vi "Drive Motor TXRX.vi"(6 "Configuration":T3={"Accelerometer Bias"={"X (m/s)"=0.0, "Y (m/s)"=0.0, "Z (m/s)"=0.0}, "Gyroscope Bias"={"X (m/s)"=0.0, "Y (m/s)"=0.0, "Z (m/s)"=0.0}, "Steering Motor Gear Ratio"=611.0, "Steering Pully Gear Ratio"=1.0, "Steering Encoder CPR"=500.0, "Steering Motor Max RPM"=4000.0, "Wheelbase (m)"=1.12, "Fork Angle (rad)"=1.3, "Balancing Controller"={"Kp (/s)"=0.0, "Kd (1)"=0.0}, "Max Allowed Steering Angle (rad)"=0.7, "Task Periods"={"Emergency Stop (us)"=0, "IMU (us)"=0, "Steering Motor Encoder (us)"=0, "State Estimator (us)"=0, "Balancing Controller (us)"=0, "GNSS (us)"=0, "Logging (us)"=0, "Drive Motor (us)"=0}, "Drive Motor Gear Ratio"=0.7}, 8 "Controller Data In":refnum<data-value>, 9 "Angular Speed (rad/s)":dbl, 10 "Drive Motor Handle In":T2, 11 "Error In":errorcluster) -> (0 "Controller Data Out":refnum<data-value>, 1 "Drive Motor Data":T1, 2 "Drive Motor Handle Out":T2, 3 "Error Out":errorcluster)   [LabVIEW 2021]
uses:
  Drive Motor Handle.ctl
  Configuration/Configuration.ctl
  Drive Motor Data.ctl
  Logging/Controller Data.ctl
  Steering Motor/Steering Motor Data.ctl
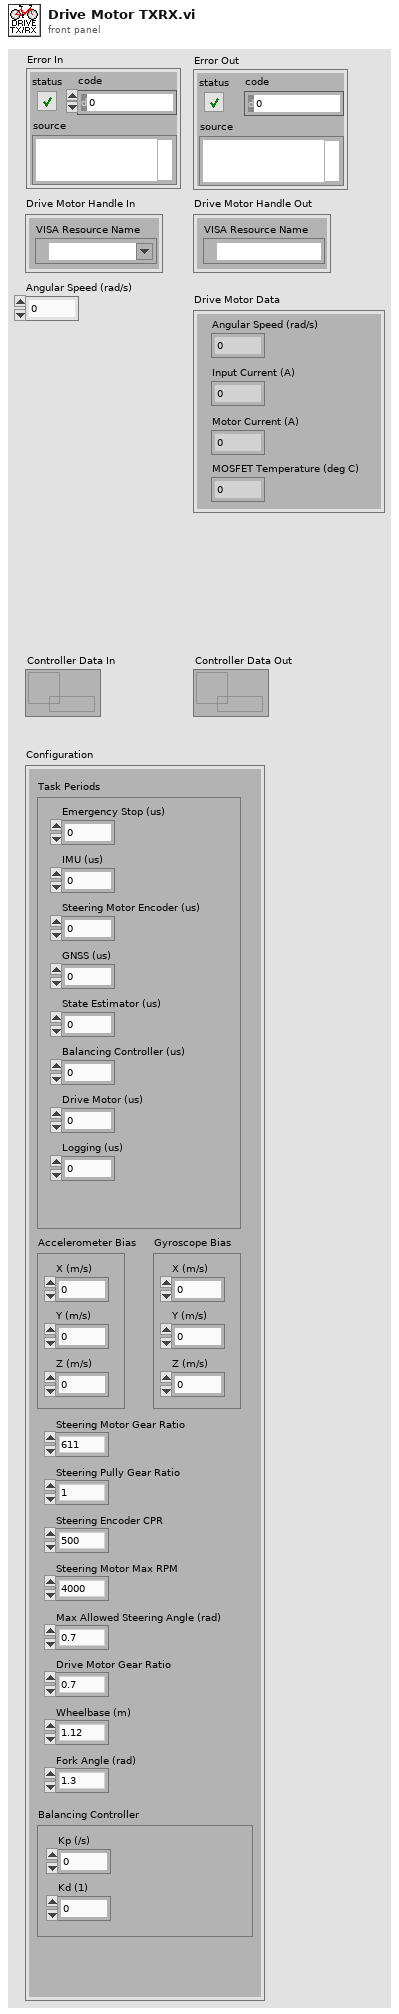
[diagram p1: front panel]
types:
  T1 = typedef "Drive Motor Data.ctl" = cluster{"Angular Speed (rad/s)":dbl, "Input Current (A)":dbl, "Motor Current (A)":dbl, "MOSFET Temperature (deg C)":dbl}
  T2 = typedef "Drive Motor Handle.ctl" = cluster{"VISA Resource Name":refnum<visa-resource-name>}
  T3 = typedef "Configuration.ctl" = cluster{"Accelerometer Bias":cluster{"X (m/s)":dbl, "Y (m/s)":dbl, "Z (m/s)":dbl}, "Gyroscope Bias":cluster{"X (m/s)":dbl, "Y (m/s)":dbl, "Z (m/s)":dbl}, "Steering Motor Gear Ratio":dbl, "Steering Pully Gear Ratio":dbl, "Steering Encoder CPR":dbl, "Steering Motor Max RPM":dbl, "Wheelbase (m)":dbl, "Fork Angle (rad)":dbl, "Balancing Controller":cluster{"Kp (/s)":dbl, "Kd (1)":dbl}, "Max Allowed Steering Angle (rad)":dbl, "Task Periods":cluster{"Emergency Stop (us)":i64, "IMU (us)":i64, "Steering Motor Encoder (us)":i64, "State Estimator (us)":i64, "Balancing Controller (us)":i64, "GNSS (us)":i64, "Logging (us)":i64, "Drive Motor (us)":i64}, "Drive Motor Gear Ratio":dbl}
  T4 = typedef "Controller Data.ctl" = cluster{"Drive Motor Data":T1, "Steering Motor Data":T5}
  T5 = typedef "Steering Motor Data.ctl" = cluster{"PWM":dbl, "Steering Angle Rate (rad/s)":dbl}
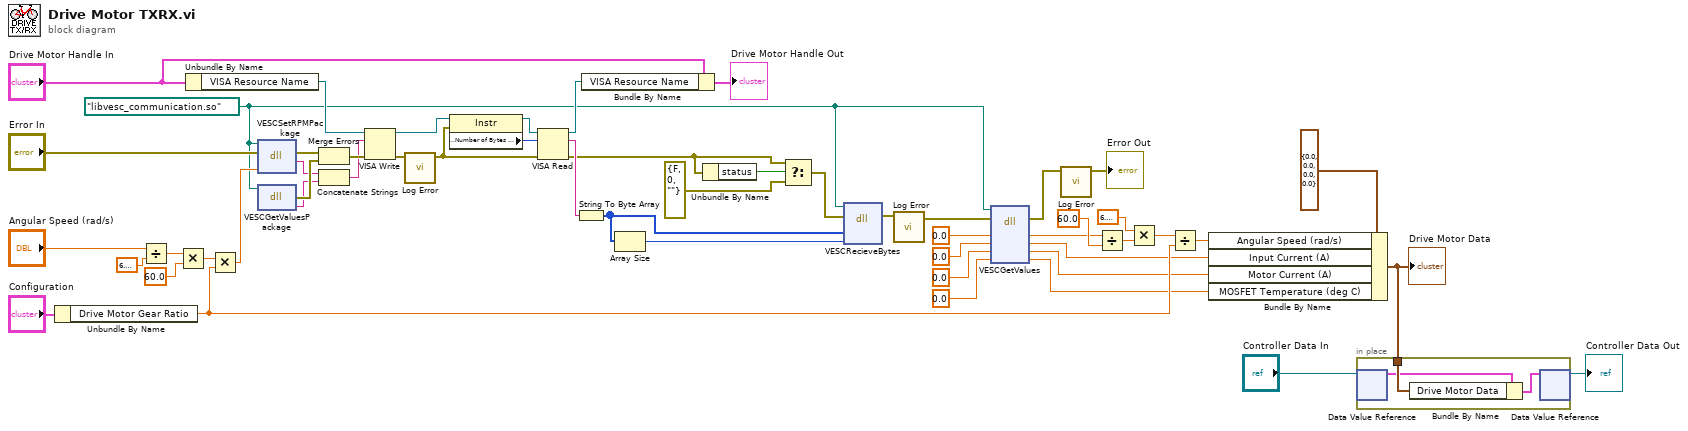
[diagram p0: block diagram]
diagram:
  w36 = path "libvesc_communication.so" ("path in")
  n1 = Unbundle By Name("Configuration") -> ("Drive Motor Gear Ratio"=w35:dbl)
  n2 = Divide(x="Angular Speed (rad/s)", y=6.283185307179586) -> (x/y=w50:dbl)
  n3 = Multiply(x=w50, y=60.0) -> (x*y=w48:dbl)
  n4 = Unbundle By Name("Drive Motor Handle In") -> ("VISA Resource Name"=w42:refnum<visa-resource-name>)
  n5 = Multiply(x=w48, y=w35) -> (x*y=w47:dbl)
  n6 = dll-call lib="?" fn="VESCSetRPMPackage"(path in=w36, error in="Error In", "RPM"=w47) -> (error out=w41:errorcluster, "Package"=w3:string)  [unwired: 2 in, 1 out]
  n7 = dll-call lib="?" fn="VESCGetValuesPackage"(path in=w36) -> (error out=w40:errorcluster, "Package"=w2:string)  [unwired: 2 in, 1 out]
  n8 = Merge Errors(w41, w40) -> (w39:errorcluster)
  n9 = Concatenate Strings(w3, w2) -> (w1:string)
  n10 = VISA Write(VISA resource name=w42, write buffer=w1, error in (no error)=w39) -> (VISA resource name out=w38:refnum<visa-resource-name>, error out=w45:errorcluster)  [unwired: 1 out]
  n11 = call "Log Error.vi"("Error In"=w45) -> ("Error Out"=w24:errorcluster)  [unwired: 10 in]
  n12 = property class="Instr"(reference=w38, error in=w24) -> (reference out=w31:refnum<visa-resource-name>, "Serial Settings:Number of Bytes at Serial Port"=w34:u32)  [unwired: 1 out]
  n13 = VISA Read(VISA resource name=w31, byte count=w34, error in (no error)=w24) -> (VISA resource name out=w37:refnum<visa-resource-name>, read buffer=w33:string, error out=w32:errorcluster)  [unwired: 1 out]
  n14 = String To Byte Array(string=w33) -> (unsigned byte array=w29:u8[])
  n15 = Bundle By Name(cluster="Drive Motor Handle In", "VISA Resource Name"=w37) -> (→"Drive Motor Handle Out":T2)
  n16 = Array Size(array=w29) -> (size(s)=w30:i32)
  n17 = Unbundle By Name(w32) -> ("status"=w28:bool)
  n18 = Select(t=w32, s=w28, f=errorcluster {"status"=FALSE, "code"=0, "source"=""}) -> (s? t:f=w27:errorcluster)
  n19 = dll-call lib="?" fn="VESCRecieveBytes"(path in=w36, error in=w27, "bytes"=w29, "length"=w30) -> (error out=w25:errorcluster)  [unwired: 4 in, 1 out]
  n20 = call "Log Error.vi"("Error In"=w25) -> ("Error Out"=w4:errorcluster)  [unwired: 10 in]
  n21 = dll-call lib="?" fn="VESCGetValues"(path in=w36, error in=w4, "RPM"=0.0, "currentIn"=0.0, "currentMotor"=0.0 ("RPM"), "tempMOS"=0.0 ("currentIn")) -> (error out=w15:errorcluster, "RPM"=w13:dbl, "currentIn"=w12:dbl, "currentMotor"=w17:dbl, "tempMOS"=w5:dbl)  [unwired: 2 in, 1 out]
  n22 = call "Log Error.vi"("Error In"=w15) -> ("Error Out"=→"Error Out":errorcluster)  [unwired: 10 in]
  n23 = Divide(x=w13, y=60.0 ("x")) -> (x/y=w19:dbl)
  n24 = Multiply(x=6.283185307179586, y=w19) -> (x*y=w11:dbl)
  n25 = Divide(x=w11, y=w35) -> (x/y=w10:dbl)
  n26 = Bundle By Name(cluster=T1 {"Angular Speed (rad/s)"=0.0, "Input Current (A)"=0.0, "Motor Current (A)"=0.0, "MOSFET Temperature (deg C)"=0.0} ("Drive Motor Data"), "Angular Speed (rad/s)"=w10, "Input Current (A)"=w12, "Motor Current (A)"=w17, "MOSFET Temperature (deg C)"=w5) -> (w7:T1)
  "Drive Motor Data" <- w7
  n27 = in-place {
    in-place-border: w7 -> [w55]
    n28 = in-place-dvr #1("Controller Data In") -> (w54:T4)  [unwired: 1 out]
    n29 = Bundle By Name(cluster=w54, "Drive Motor Data"=w55) -> (w56:T4)
    n30 = in-place-dvr #1(w56) -> (→"Controller Data Out":refnum<data-value>)  [unwired: 1 out]
  }
